vi "DesiredBundle2DesiredRow.vi"(0 "DesiredParameters":T1, 7 "CMD Step":dbl format="%#_13g") -> (4 "DesiredStatRow":string[](array[string]))   [LabVIEW 2013]
uses:
  TypeDef/Command Cluster.ctl
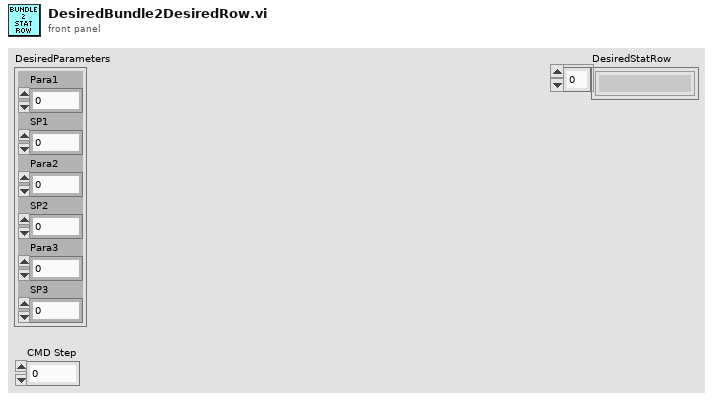
[diagram p1: front panel]
types:
  T1 = typedef "Command Cluster.ctl" = cluster{"Para1":i32, "SP1":dbl, "Para2":i32, "SP2":dbl, "Para3":i32, "SP3":dbl}
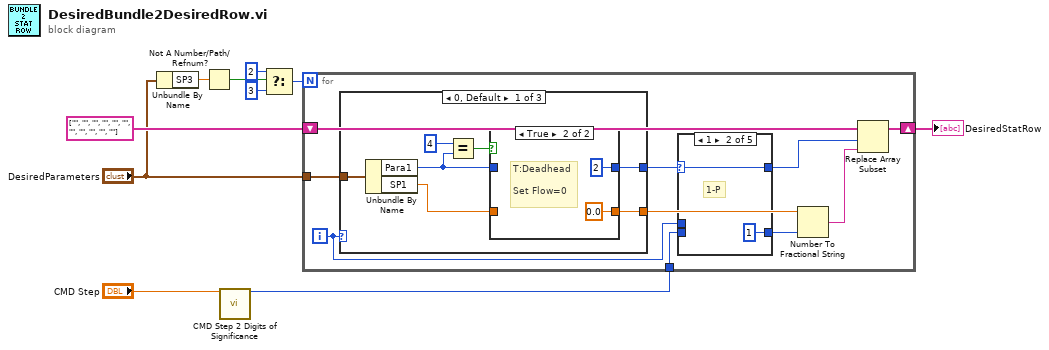
[diagram p0: block diagram]
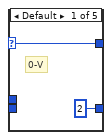
[diagram p2: hidden frame]
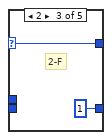
[diagram p3: hidden frame]
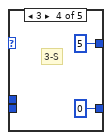
[diagram p4: hidden frame]
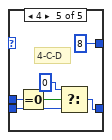
[diagram p5: hidden frame]
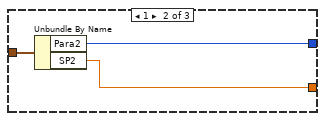
[diagram p7: hidden frame]
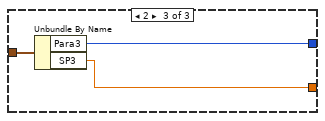
[diagram p8: hidden frame]
diagram:
  n1 = Unbundle By Name("DesiredParameters") -> ("SP3"=w2:dbl)
  n2 = Not A Number/Path/Refnum?(number/path/refnum=w2) -> (NaN/Path/Refnum?=w1:bool)
  n3 = call "CMD Step 2 Digits of Significance.vi"("CMD Step"="CMD Step") -> ("Digits of Significance"=w7:i32)  [unwired: 14 in]
  n4 = Select(t=2, s=w1, f=3) -> (s? t:f=w3:i32)
  n5 = for {
    N: w3 -> [_]
    tunnel: "DesiredParameters" -> [w20]
    shift-right: [w18] -> w9
    shift-left: string[] ["", "", "", "", "", "", "", "", "", "", ""] -> [w19]
    tunnel: w7 -> [w12]
    i -> [w11]
    n6 = case shown="0, Default" w11 {
      tunnel: w20 -> [w41 w48 w51]
      tunnel: [w35 w47 w50] -> w15
      tunnel: [w36 w46 w49] -> w17
      frame 0, Default {
        n7 = Unbundle By Name(w41) -> ("Para1"=w37:i32, "SP1"=w38:dbl)
        n8 = Equal?(x=4, y=w37) -> (x = y?=w39:bool)
        n9 = case shown="True" w39 {
          tunnel: w38 -> [w42 _]
          tunnel: w37 -> [w43 _]
          tunnel: [w43 2 ("Para1")] -> w36
          tunnel: [w42 0.0 ("SP1")] -> w35
          frame False {
          }
          frame True {
            # "T:Deadhead\n\nSet Flow=0"
          }
        }
      }
      frame 1 {
        n10 = Unbundle By Name(w48) -> ("Para2"=w46:i32, "SP2"=w47:dbl)
      }
      frame 2 {
        n11 = Unbundle By Name(w51) -> ("Para3"=w49:i32, "SP3"=w50:dbl)
      }
    }
    n12 = case shown="1" w17 {
      selector: w17 -> [w22 w24 w26 _ _]
      tunnel: [w22 w24 w26 5 ("Para1") 8 ("Para1")] -> w16
      tunnel: [2 1 1 0 w30] -> w13
      tunnel: w12 -> [_ _ _ _ w31]
      tunnel: w11 -> [_ _ _ _ w33]
      frame Default {
        # "0-V"
      }
      frame 1 {
        # "1-P"
      }
      frame 2 {
        # "2-F"
      }
      frame 3 {
        # "3-S"
      }
      frame 4 {
        # "4-C-D"
        n13 = Equal To 0?(x=w33) -> (x = 0?=w32:bool)
        n14 = Select(t=0, s=w32, f=w31) -> (s? t:f=w30:i32)
      }
    }
    n15 = Number To Fractional String(number=w15, precision (6)=w13) -> (F-format string=w14:string)  [unwired: 2 in]
    n16 = Replace Array Subset(array=w19, new element=w14, index=w16) -> (w18:string[])
  }
  "DesiredStatRow" <- w9
